vi "UDP_Read_string.vi"() -> ()   [LabVIEW 2014]
panel:
  in  "stop":bool
  out "String":string
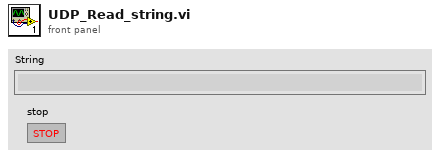
[diagram p1: front panel]
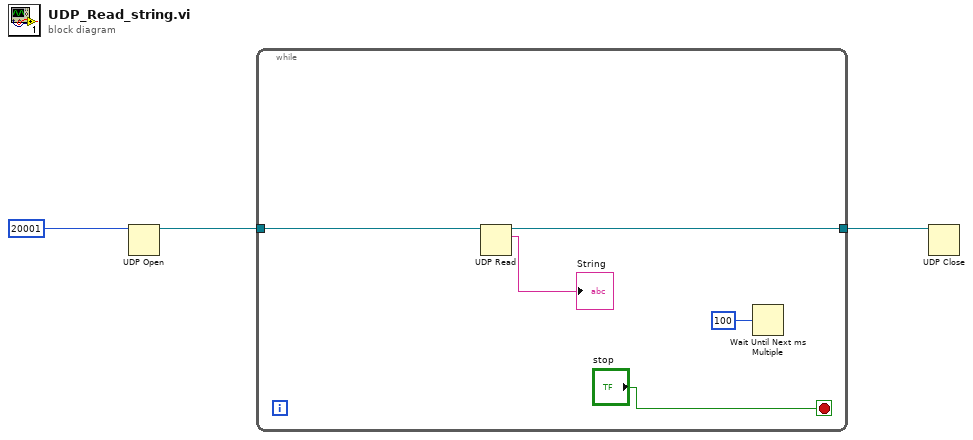
[diagram p0: block diagram]
diagram:
  n1 = UDP Open(11:u16 20001 ("port")) -> (port=w2:refnum<k16>)  [unwired: 4 in, 2 out]
  n2 = while {
    tunnel: w2 -> [w8]
    tunnel: [w7] -> w1
    stop <- "stop" stop-if-true
    n3 = UDP Read(connection ID=w8) -> (data out=→"String":string, 3:w7:refnum<k16>)  [unwired: 3 in, 3 out]
    n4 = Wait Until Next ms Multiple(millisecond multiple=u32 100) -> ()  [unwired: 1 out]
  }
  n5 = UDP Close(connection ID=w1) -> ()  [unwired: 1 in, 2 out]
